vi "Stop Measurements.vi"(8 "error in (no error)":errorcluster, 11 "Measure Controller in":refnum<class "Measure Controller.lvclass">) -> (0 "error out":errorcluster, 3 "Measure Controller out":refnum<class "Measure Controller.lvclass">)   [LabVIEW 2015, in "Measure Controller.lvclass"]
uses:
  Measure Controller.lvclass
  Measure Controller.lvclass/Measure Controller.ctl
  <vilib>/ActorFramework/Message Enqueuer/Message Enqueuer.lvclass/Message Enqueuer.ctl
  Read Active measurements enqueuers.vi
  <vilib>/ActorFramework/Message Enqueuer/Enqueue.vi
  <vilib>/ActorFramework/Message Priority Queue/Priority Enqueue.vi
  <vilib>/ActorFramework/Message Enqueuer/Message Enqueuer.lvclass
  Measure Object Messages/Stop Acquire Msg/Stop Acquire Msg.lvclass
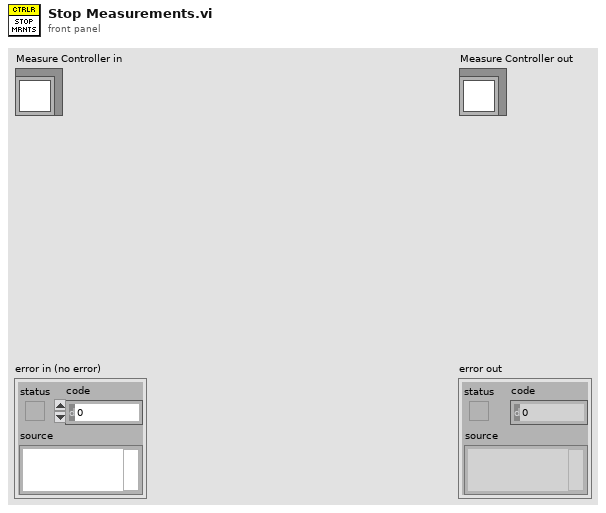
[diagram p1: front panel]
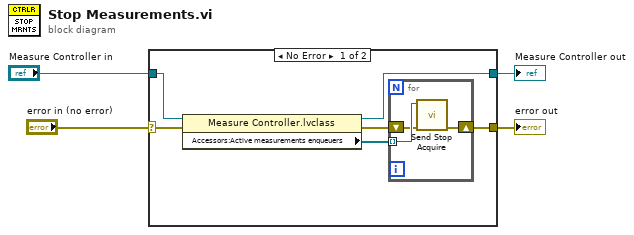
[diagram p0: block diagram]
diagram:
  n1 = case shown="No Error" "error in (no error)" {
    selector: "error in (no error)" -> [w6 w15]
    tunnel: [w5 w15] -> w3
    tunnel: [w9 w14] -> w1
    tunnel: "Measure Controller in" -> [w10 w14]
    frame No Error {
      n2 = property class="Measure Controller.lvclass"(reference=w10, error in=w6) -> (reference out=w9:refnum<class "Measure Controller.lvclass">, error out=w7:errorcluster, "Accessors:Active measurements enqueuers"=w8:refnum<class "Message Enqueuer.lvclass">[])
      n3 = for {
        tunnel: w8 -> [w13] mode=indexing
        shift-right: [w11] -> w5
        shift-left: w7 -> [w12]
        n4 = call "Send Stop Acquire.vi"("error in (no error)"=w12, "Message Enqueuer"=w13) -> ("error out"=w11:errorcluster)  [unwired: 8 in, 1 out]
      }
    }
    frame Error {
    }
  }
  "error out" <- w3
  "Measure Controller out" <- w1
